vi "Table - Justify.vi"(7 "Col Header Justification (Center)":enum16{"Left", "Center", "Right"}(ring)=enum."Center", 8 "error in":errorcluster, 9 "Row Header Justification (Left)":enum16{"Left", "Center", "Right"}(ring), 10 "Data Justification (center)":enum16{"Left", "Center", "Right"}(ring)=enum."Center", 11 "Table":refnum<vi>) -> (0 "error out":errorcluster)   [LabVIEW 2015, in "Utility.lvlib"]
uses:
  Utility.lvlib
  <vilib>/Utility/miscctls.llb/LVRowAndColumnTypeDef.ctl
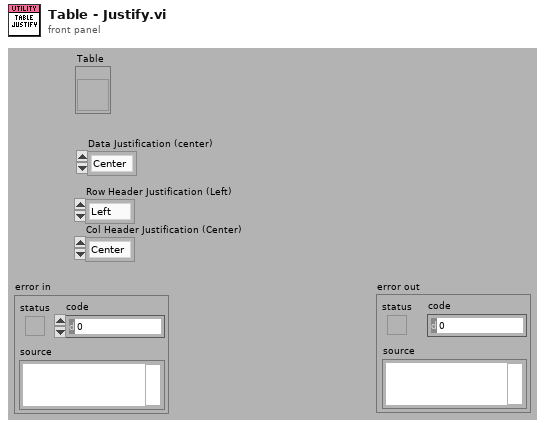
[diagram p1: front panel]
types:
  T1 = typedef "LVRowAndColumnTypeDef.ctl" = cluster{"Row":i32, "Column":i32}
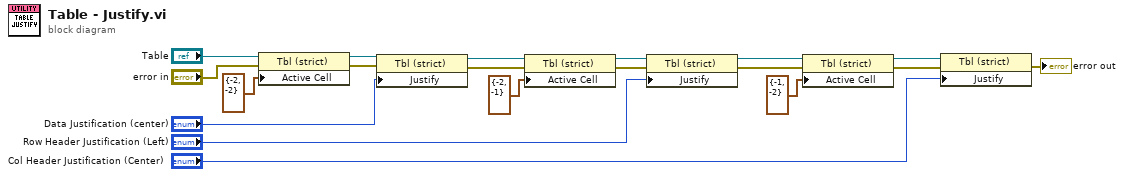
[diagram p0: block diagram]
diagram:
  n1 = property class="Tbl (strict)"(reference="Table", error in="error in", "Active Cell"=T1 {"Row"=-2, "Column"=-2} ("Edit Position")) -> (reference out=w12:refnum<vi>, error out=w7:errorcluster)
  n2 = property class="Tbl (strict)"(reference=w12, error in=w7, "Justify"="Data Justification (center)") -> (reference out=w17:refnum<vi>, error out=w6:errorcluster)
  n3 = property class="Tbl (strict)"(reference=w17, error in=w6, "Active Cell"=T1 {"Row"=-2, "Column"=-1} ("Edit Position")) -> (reference out=w16:refnum<vi>, error out=w5:errorcluster)
  n4 = property class="Tbl (strict)"(reference=w16, error in=w5, "Justify"="Row Header Justification (Left)") -> (reference out=w9:refnum<vi>, error out=w4:errorcluster)
  n5 = property class="Tbl (strict)"(reference=w9, error in=w4, "Active Cell"=T1 {"Row"=-1, "Column"=-2} ("Edit Position")) -> (reference out=w10:refnum<vi>, error out=w3:errorcluster)
  n6 = property class="Tbl (strict)"(reference=w10, error in=w3, "Justify"="Col Header Justification (Center)") -> (error out=→"error out":errorcluster)  [unwired: 1 out]
